vi "Get Process Classes.vi"(8 "error in (no error)":errorcluster, 11 "New Class Dialog In":refnum<class "New Class Dialog.lvclass">) -> (0 "error out":errorcluster, 3 "New Class Dialog Out":refnum<class "New Class Dialog.lvclass">)   [LabVIEW 2020, in "Process Generation.lvlib" / "New Class Dialog.lvclass"]
uses:
  New Class Dialog.lvclass
  Framework/Application/Application.lvclass
  C:/Git/astemes-triarc-framework/source/Framework/Process/Process.lvclass
  Framework/View/View.lvclass
  Framework/Process/Process.lvclass
  New Class Dialog.lvclass/New Class Dialog.ctl
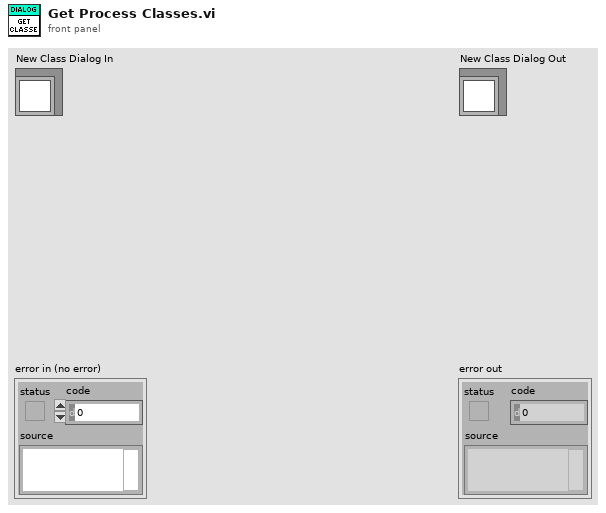
[diagram p1: front panel]
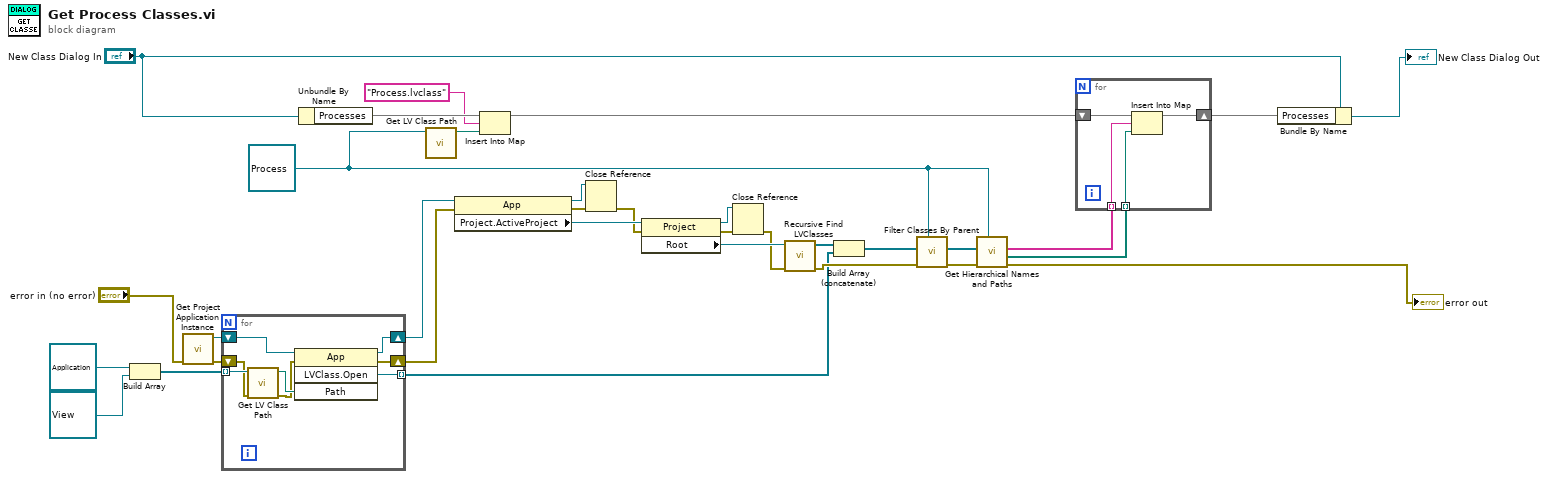
[diagram p0: block diagram]
diagram:
  w1 = refnum<class "Process.lvclass"> refnum ("Process.lvclass")
  n1 = Build Array(refnum<class "Application.lvclass"> refnum ("Application.lvclass"), refnum<class "View.lvclass"> refnum ("View.lvclass")) -> (w20:refnum<class "Process.lvclass">[])
  n2 = call "Get Project Application Instance.vi"("error in (no error)"="error in (no error)") -> ("error out"=w17:errorcluster, "Application out"=w16:refnum<vi>)  [unwired: 9 in]
  n3 = for {
    tunnel: w20 -> [w41] mode=indexing
    tunnel: [w39] -> w18 mode=indexing
    shift-right: [w37] -> w13
    shift-left: w16 -> [w36]
    shift-right: [w35] -> w14
    shift-left: w17 -> [w34]
    n4 = call <vilib>:"Get LV Class Path.vi"("error in (no error)"=w34, "object"=w41) -> ("error out"=w38:errorcluster, "class path"=w40:path)  [unwired: 8 in]
    n5 = invoke class="App" method="LVClass.Open"(reference=w36, error in=w38, "Path"=w40) -> (reference out=w37:refnum<vi>, error out=w35:errorcluster, "LVClass.Open"=w39:refnum<vi>)  [unwired: 1 in, 1 out]
  }
  n6 = Unbundle By Name("New Class Dialog In") -> ("Processes"=w33:map{string, path})
  n7 = call <vilib>:"Get LV Class Path.vi"("object"=w1) -> ("class path"=w11:path)  [unwired: 9 in, 1 out]
  n8 = property class="App"(reference=w13, error in=w14) -> (reference out=w23:refnum<vi>, error out=w25:errorcluster, "Project.ActiveProject"=w26:refnum<vi>)
  n9 = Insert Into Map(map in=w33, key="Process.lvclass", value=w11) -> (map out=w7:map{string, path})  [unwired: 2 out]
  n10 = Close Reference(reference=w23, error in (no error)=w25) -> (error out=w24:errorcluster)
  n11 = property class="Project"(reference=w26, error in=w24) -> (reference out=w32:refnum<vi>, error out=w31:errorcluster, "Root"=w30:refnum<vi>)
  n12 = Close Reference(reference=w32, error in (no error)=w31) -> (error out=w29:errorcluster)
  n13 = call "Recursive Find LVClasses.vi"("error in (no error)"=w29, "reference"=w30) -> ("error out"=w28:errorcluster, "Class References"=w27:refnum<vi>[])  [unwired: 8 in]
  n14 = Build Array (concatenate)(w27, w18) -> (w19:refnum<vi>[])
  n15 = call "Filter Classes By Parent.vi"("Parent Class"=w1, "error in (no error)"=w28, "Class References"=w19) -> ("error out"=w10:errorcluster, "Class References"=w8:refnum<vi>[])  [unwired: 7 in]
  n16 = call "Get Hierarchical Names and Paths.vi"("Parent Class"=w1, "error in (no error)"=w10, "Class References"=w8) -> ("error out"=→"error out":errorcluster, "Paths"=w6:path[], "Names"=w5:string[])  [unwired: 6 in]
  n17 = for {
    shift-right: [w44] -> w3
    shift-left: w7 -> [w45]
    tunnel: w6 -> [w43] mode=indexing
    tunnel: w5 -> [w42] mode=indexing
    n18 = Insert Into Map(map in=w45, key=w42, value=w43) -> (map out=w44:map{string, path})  [unwired: 2 out]
  }
  n19 = Bundle By Name(cluster="New Class Dialog In", "Processes"=w3) -> (→"New Class Dialog Out":refnum<class "New Class Dialog.lvclass">)
